vi "CupFinderV4.vi"() -> ()   [LabVIEW 2017]
panel:
  out "WORK FOR GODS SAKE 2":T1(plugin-control)
  out "Height Ratio":dbl
  in  "stop":bool
  out "Y-Out":dbl
  out "X-Out":dbl
  out "CupPosition":T1(plugin-control)
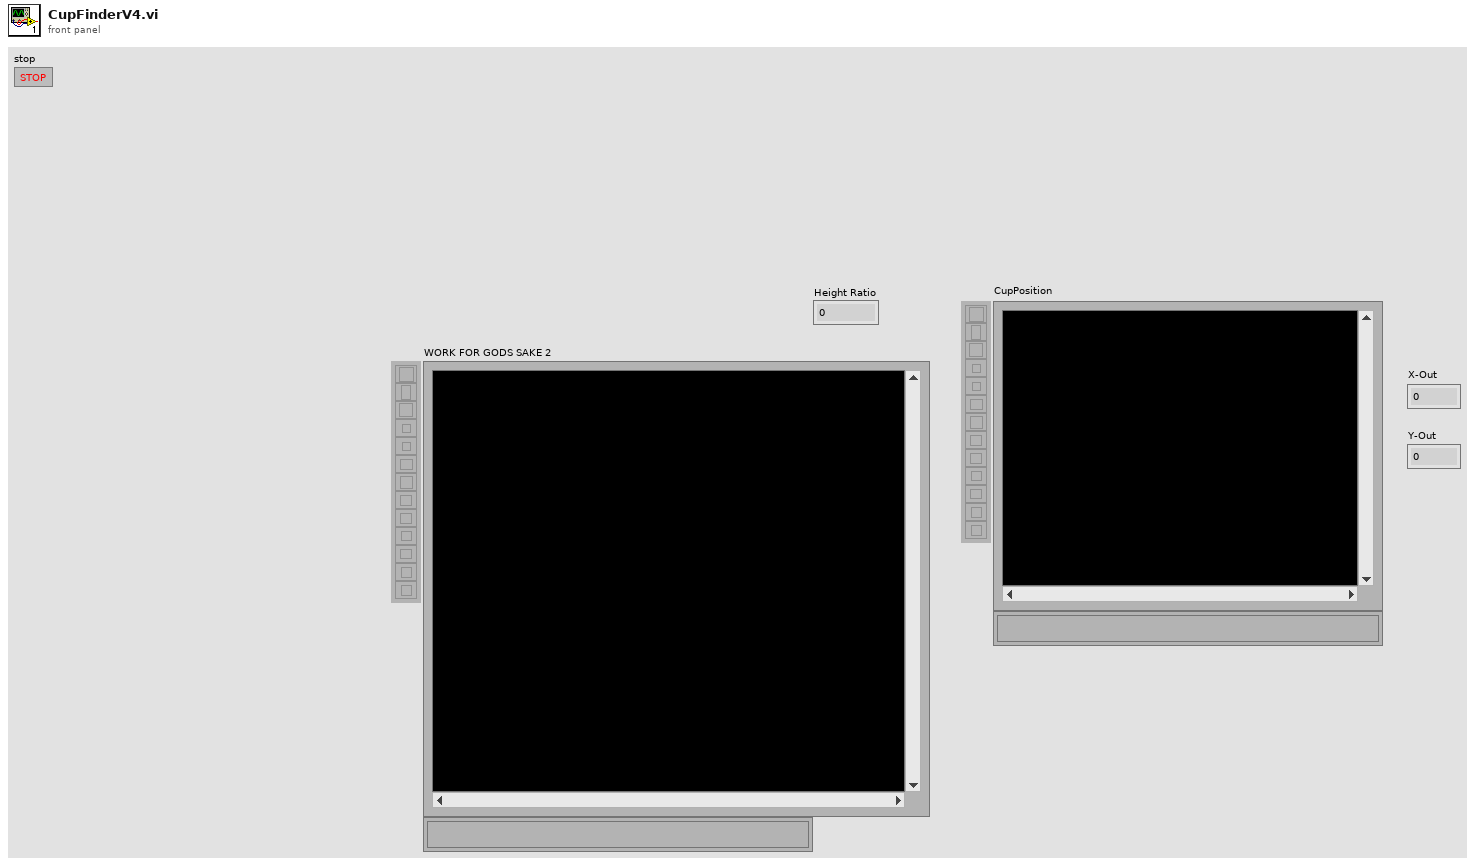
[diagram p1: front panel]
types:
  T1 = typedef "IMAQ Image.ctl" = refnum<image>
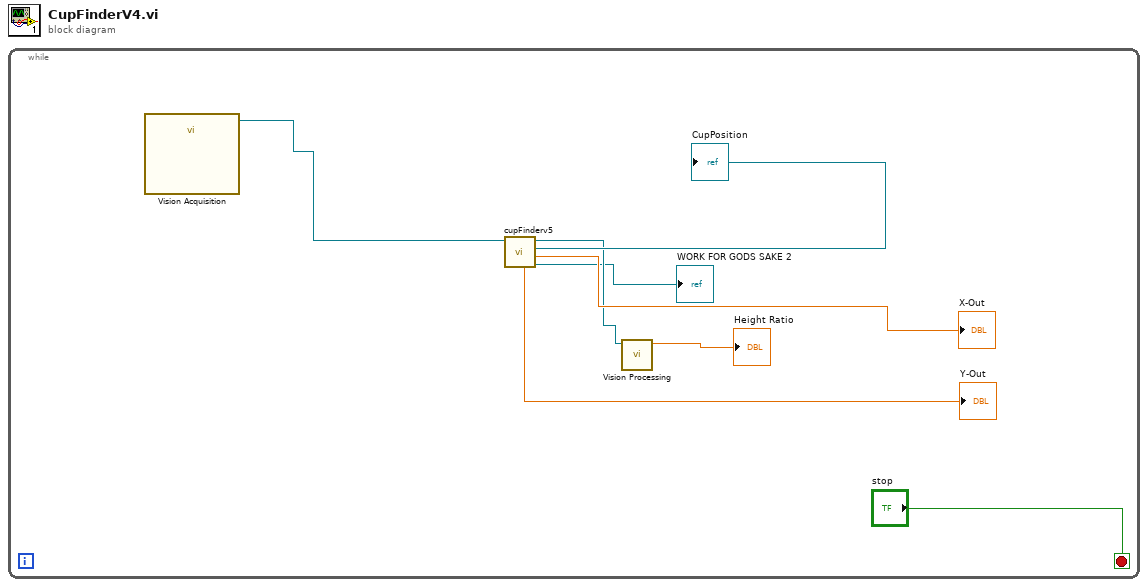
[diagram p0: block diagram]
diagram:
  n1 = while {
    stop <- "stop" stop-if-true
    n2 = call "Vision Acquisition"() -> ("Image Out"=w5:T1)  [unwired: 25 in, 2 out]
    n3 = call "cupFinderv5.vi"("image\n in"=w5) -> ("WORK FOR GODS SAKE 2"=→"WORK FOR GODS SAKE 2":T1, "X-Out"=→"X-Out":dbl, "CupPosition"=→"CupPosition":T1, "Refnum out"=w3:T1, "Y-Out"=→"Y-Out":dbl)  [unwired: 5 in, 1 out]
    n4 = call "Vision Processing.vi"("Image In"=w3) -> ("Height Ratio"=→"Height Ratio":dbl)  [unwired: 10 in]
  }
